vi "Get Error Codes.vi"(8 "error in (no error)":errorcluster, 11 "RS-xxx to GPIB ConvBox in":refnum<class "RS-xxx to GPIB ConvBox.lvclass">) -> (0 "error out":errorcluster, 2 "Error Codes":cluster{"Code":i32, "String":string}[](array[cluster]), 3 "RS-xxx to GPIB ConvBox out":refnum<class "RS-xxx to GPIB ConvBox.lvclass">)   [LabVIEW 2019, in "Protocols.lvlib" / "RS-xxx to GPIB ConvBox.lvclass"]
uses:
  RS-xxx to GPIB ConvBox.lvclass
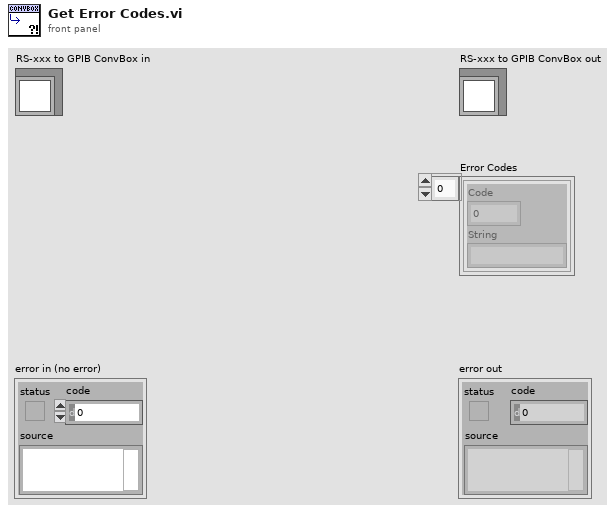
[diagram p1: front panel]
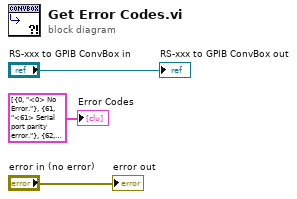
[diagram p0: block diagram]
diagram:
  "error out" <- "error in (no error)"
  "RS-xxx to GPIB ConvBox out" <- "RS-xxx to GPIB ConvBox in"
  "Error Codes" <- cluster{"Code":i32, "String":string}[] [{"Code"=0, "String"="<0> No Error."}, {"Code"=61, "String"="<61> Serial port parity error."}, {"Code"=62, "String"="<62> Serial port overrun error."}, {"Code"=63, "String"="<63> Serial port receive buffer overflow."}, {"Code"=64, "String"="<64> Serial port framing error."}, {"Code"=65, "String"="<65> Serial port timeout; bytes not received at serial port."}, {"Code"=-1073807360, "String"="<-1073807360> Unknown system error (miscellaneous error)."}, {"Code"=-1073807346, "String"="<-1073807346> The given session or object reference is invalid."}, {"Code"=-1073807345, "String"="<-1073807345> Specified type of lock cannot be obtained, or specified operation cannot be performed, because the resource is locked."}, {"Code"=-1073807344, "String"="<-1073807344> Invalid expression specified for search."}, {"Code"=-1073807343, "String"="<-1073807343> Insufficient location information or the device or resource is not present in the system."}, {"Code"=-1073807342, "String"="<-1073807342> Invalid resource reference specified. Parsing error."}, {"Code"=-1073807341, "String"="<-1073807341> Invalid access mode."}, {"Code"=-1073807339, "String"="<-1073807339> Timeout expired before operation completed."}, {"Code"=-1073807338, "String"="<-1073807338> The VISA driver failed to properly close the session or object reference."}, {"Code"=-1073807333, "String"="<-1073807333> Specified degree is invalid."}, {"Code"=-1073807332, "String"="<-1073807332> Specified job identifier is invalid."}, {"Code"=-1073807331, "String"="<-1073807331> The specified attribute is not defined or supported by the referenced resource."}, {"Code"=-1073807330, "String"="<-1073807330> The specified state of the attribute is not valid, or is not supported as defined by the resource."}, {"Code"=-1073807329, "String"="<-1073807329> The specified attribute is read-only."}, {"Code"=-1073807328, "String"="<-1073807328> The specified type of lock is not supported by this resource."}, {"Code"=-1073807327, "String"="<-1073807327> The access key to the specified resource is invalid."}, {"Code"=-1073807322, "String"="<-1073807322> Specified event type is not supported by the resource."}, {"Code"=-1073807321, "String"="<-1073807321> Invalid mechanism specified."}, {"Code"=-1073807320, "String"="<-1073807320> A handler was not installed."}, {"Code"=-1073807319, "String"="<-1073807319> The given handler reference is invalid."}, {"Code"=-1073807318, "String"="<-1073807318> Specified event context is invalid."}, {"Code"=-1073807315, "String"="<-1073807315> The event queue for the specified type has overflowed."}, {"Code"=-1073807313, "String"="<-1073807313> You must be enabled for events of the specified type in order to receive them."}, {"Code"=-1073807312, "String"="<-1073807312> User abort occurred during transfer."}, {"Code"=-1073807308, "String"="<-1073807308> Violation of raw write protocol occurred during transfer."}, {"Code"=-1073807307, "String"="<-1073807307> Violation of raw read protocol occurred during transfer."}, {"Code"=-1073807306, "String"="<-1073807306> Device reported an output protocol error during transfer."}, {"Code"=-1073807305, "String"="<-1073807305> Device reported an input protocol error during transfer."}, {"Code"=-1073807304, "String"="<-1073807304> Bus error occurred during transfer."}, {"Code"=-1073807303, "String"="<-1073807303> Unable to queue the asynchronous operation because there is already an operation in progress."}, {"Code"=-1073807302, "String"="<-1073807302> Unable to start operation because setup is invalid (due to attributes being set to an inconsistent state)."}, {"Code"=-1073807301, "String"="<-1073807301> Unable to queue the asynchronous operation."}, {"Code"=-1073807300, "String"="<-1073807300> Insufficient system resources to perform necessary memory allocation."}, {"Code"=-1073807299, "String"="<-1073807299> Invalid buffer mask specified."}, {"Code"=-1073807298, "String"="<-1073807298> Could not perform operation because of I/O error."}, {"Code"=-1073807297, "String"="<-1073807297> A format specifier in the format string is invalid."}, {"Code"=-1073807295, "String"="<-1073807295> A format specifier in the format string is not supported."}, {"Code"=-1073807294, "String"="<-1073807294> The specified trigger line is currently in use."}, {"Code"=-1073807290, "String"="<-1073807290> The specified mode is not supported by this VISA implementation."}, {"Code"=-1073807286, "String"="<-1073807286> Service request has not been received for the session."}, {"Code"=-1073807282, "String"="<-1073807282> Invalid address space specified."}, {"Code"=-1073807279, "String"="<-1073807279> Invalid offset specified."}, {"Code"=-1073807278, "String"="<-1073807278> Invalid access width specified."}, {"Code"=-1073807276, "String"="<-1073807276> Specified offset is not accessible from this hardware."}, {"Code"=-1073807275, "String"="<-1073807275> Cannot support source and destination widths that are different."}, {"Code"=-1073807273, "String"="<-1073807273> The specified session is not currently mapped."}, {"Code"=-1073807271, "String"="<-1073807271> A previous response is still pending, causing a multiple query error."}, {"Code"=-1073807265, "String"="<-1073807265> No listeners condition is detected (both NRFD and NDAC are deasserted)."}, {"Code"=-1073807264, "String"="<-1073807264> The interface associated with this session is not currently the controller in charge."}, {"Code"=-1073807263, "String"="<-1073807263> The interface associated with this session is not the system controller."}, {"Code"=-1073807257, "String"="<-1073807257> The given session or object reference does not support this operation."}, {"Code"=-1073807256, "String"="<-1073807256> An interrupt is still pending from a previous call."}, {"Code"=-1073807254, "String"="<-1073807254> A parity error occurred during transfer."}, {"Code"=-1073807253, "String"="<-1073807253> A framing error occurred during transfer."}, {"Code"=-1073807252, "String"="<-1073807252> An overrun error occurred during transfer."}, {"Code"=-1073807250, "String"="<-1073807250> The path from trigSrc to trigDest is not currently mapped."}, {"Code"=-1073807248, "String"="<-1073807248> The specified offset is not properly aligned for the access width of the operation."}, {"Code"=-1073807247, "String"="<-1073807247> A specified user buffer is not valid or cannot be accessed for the required size."}, {"Code"=-1073807246, "String"="<-1073807246> The resource is valid, but VISA cannot currently access it."}, {"Code"=-1073807242, "String"="<-1073807242> Specified width is not supported by this hardware."}, {"Code"=-1073807240, "String"="<-1073807240> The value of some parameter (which parameter is not known) is invalid."}, {"Code"=-1073807239, "String"="<-1073807239> The protocol specified is invalid."}, {"Code"=-1073807237, "String"="<-1073807237> Invalid size of window specified."}, {"Code"=-1073807232, "String"="<-1073807232> The specified session currently contains a mapped window."}, {"Code"=-1073807231, "String"="<-1073807231> The given operation is not implemented."}, {"Code"=-1073807229, "String"="<-1073807229> Invalid length specified."}, {"Code"=-1073807215, "String"="<-1073807215> Invalid mode specified."}, {"Code"=-1073807204, "String"="<-1073807204> The current session did not have a lock on the resource."}, {"Code"=-1073807202, "String"="<-1073807202> VISA or a code library required by VISA could not be located or loaded."}, {"Code"=-1073807201, "String"="<-1073807201> The interface cannot generate an interrupt on the requested level or with the requested statusID value."}, {"Code"=-1073807200, "String"="<-1073807200> The value specified by the line parameter is invalid."}, {"Code"=-1073807199, "String"="<-1073807199> An error occurred while trying to open the specified file. Possible reasons include an invalid path or lack of access rights."}, {"Code"=-1073807198, "String"="<-1073807198> An error occurred while performing I/O on the specified file."}, {"Code"=-1073807197, "String"="<-1073807197> One of the specified lines, trigSrc or trigDest, is not supported by this VISA implementation, or the combination of lines is not a valid mapping."}, {"Code"=-1073807196, "String"="<-1073807196> The specified mechanism is not supported for the given event type."}, {"Code"=-1073807195, "String"="<-1073807195> The interface type is valid, but the specified interface number is not configured."}, {"Code"=-1073807194, "String"="<-1073807194> The connection for the given session has been lost."}, {"Code"=-1073807193, "String"="<-1073807193> The remote machine does not exist or is not accepting any connections."}, {"Code"=-1073807192, "String"="<-1073807192> Access to the resource or remote machine is denied. This is due to lack of sufficient privileges for the current user or machine."}, {"Code"=1073676290, "String"="<1073676290> Specified event is already enabled for at least one of the specified mechanisms."}, {"Code"=1073676291, "String"="<1073676291> Specified event is already disabled for at least one of the specified mechanisms."}, {"Code"=1073676292, "String"="<1073676292> Operation completed successfully, but queue was already empty."}, {"Code"=1073676293, "String"="<1073676293> The specified termination character was read."}, {"Code"=1073676294, "String"="<1073676294> The number of bytes transferred is equal to the requested input count. More data might be available."}, {"Code"=1073676300, "String"="<1073676300> VISA received more event information of the specified type than the configured queue size could hold."}, {"Code"=1073676407, "String"="<1073676407> The specified configuration either does not exist or could not be loaded. VISA-specified defaults will be used."}, {"Code"=1073676413, "String"="<1073676413> Session opened successfully, but the device at the specified address is not responding."}, {"Code"=1073676414, "String"="<1073676414> The path from trigSrc to trigDest is already mapped."}, {"Code"=1073676416, "String"="<1073676416> Wait terminated successfully on receipt of an event notification."}, {"Code"=1073676418, "String"="<1073676418> The specified object reference is uninitialized."}, {"Code"=1073676420, "String"="<1073676420> Although the specified state of the attribute is valid, it is not supported by this resource implementation."}, {"Code"=1073676421, "String"="<1073676421> The status code passed to the operation could not be interpreted."}, {"Code"=1073676424, "String"="<1073676424> The specified I/O buffer is not supported."}, {"Code"=1073676440, "String"="<1073676440> Event handled successfully. Do not invoke any other handlers on this session for this event."}, {"Code"=1073676441, "String"="<1073676441> Operation completed successfully, and this session has nested shared locks."}, {"Code"=1073676442, "String"="<1073676442> Operation completed successfully, and this session has nested exclusive locks."}, {"Code"=1073676443, "String"="<1073676443> Operation completed successfully, but the operation was actually synchronous rather than asynchronous."}, {"Code"=1073676457, "String"="<1073676457> The operation succeeded, but a lower level driver did not implement the extended functionality."}, {"Code"=-1073807202, "String"="<-1073807202> VISA or a code library required by VISA could not be located or loaded."}] ("appended array")
